vi "GetDefaultHistoryRate.vi"(2 "error in (no error)":errorcluster) -> (0 "error out":errorcluster, 1 "HistoryRate":i32)   [LabVIEW 2018, in "feGEM DataPacker.lvlib"]
uses:
  feGEM DataPacker.lvlib
  DataPacker/Utilities/PeriodicEnumTypeDef.ctl
panel:
  out "Periodic Tasks":string[](array[string])
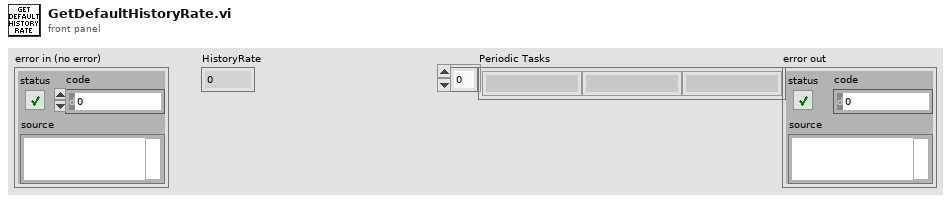
[diagram p1: front panel]
types:
  T1 = typedef "feGEM DataPacker.lvlib/PeriodicEnumTypeDef.ctl" = enum16{"GET_STATUS", "GET_HIST_RATE", "GET_RUNNO", "GET_RUN_START_T", "GET_RUN_STOP_T", "GET_TIME"}
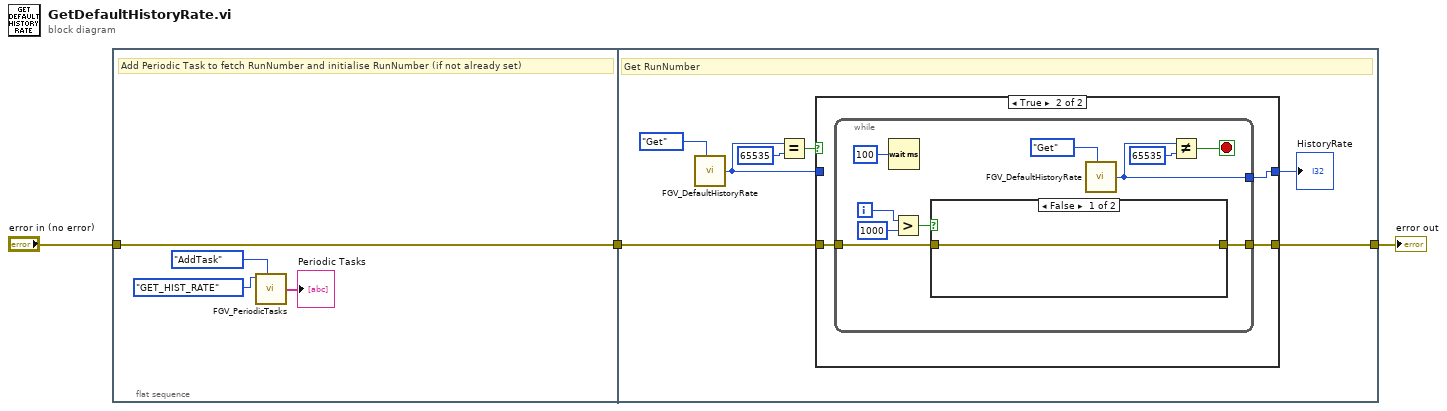
[diagram p0: block diagram]
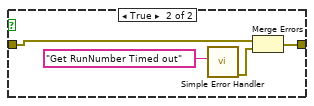
[diagram p3: hidden frame]
diagram:
  n1 = flat-sequence {
    tunnel: "error in (no error)" -> [w6]
    tunnel: [w6] -> w2
    tunnel: w2 -> [w13]
    tunnel: [w12] -> w1
    frame #0 {
      # "Add Periodic Task to fetch RunNumber and initialise RunNumber (if not already set)"
      n2 = call "FGV_PeriodicTasks.vi"("MIDAS Commands"=PeriodicEnumTypeDef."GET_HIST_RATE", "Task"=enum16{"AddTask", "GetTasks", "ClearTasks"}."AddTask") -> ("Tasks"=→"Periodic Tasks":string[])  [unwired: 3 in]
    }
    frame #1 {
      # "Get RunNumber"
      n3 = call "FGV_DefaultHistoryRate.vi"("Enum"=enum16{"Set", "Get"}."Get") -> ("Default History Rate"=w10:i32)  [unwired: 4 in]
      n4 = Equal?(x=w10, y=65535) -> (x = y?=w8:bool)
      n5 = case shown="True" w8 {
        tunnel: [w16 w19] -> w14
        tunnel: w10 -> [w16 _]
        tunnel: w13 -> [w15 w18]
        tunnel: [w15 w17] -> w12
        frame False {
        }
        frame True {
          n6 = while {
            tunnel: [w21] -> w19
            tunnel: w18 -> [w25]
            tunnel: [w24] -> w17
            i -> [w27]
            stop <- w22 stop-if-true
            n7 = Wait (ms)(milliseconds to wait=u32 100) -> ()  [unwired: 1 out]
            n8 = Greater?(x=w27, y=1000) -> (0:w26:bool)
            n9 = case shown="False" w26 {
              tunnel: w25 -> [w30 w33]
              tunnel: [w30 w31] -> w24
              frame False {
              }
              frame True {
                n10 = call <vilib>:"Simple Error Handler.vi"("error source (\" \")"="Get RunNumber Timed out" ("error source (\" \")")) -> ("error out"=w32:errorcluster)  [unwired: 4 in, 4 out]
                n11 = Merge Errors(w33, w32) -> (w31:errorcluster)
              }
            }
            n12 = call "FGV_DefaultHistoryRate.vi"("Enum"=enum16{"Set", "Get"}."Get") -> ("Default History Rate"=w21:i32)  [unwired: 4 in]
            n13 = Not Equal?(x=w21, y=65535) -> (x != y?=w22:bool)
          }
        }
      }
      "HistoryRate" <- w14
    }
  }
  "error out" <- w1
